vi "Replace Constant in VI (Scalar).vi"(8 "error in":errorcluster, 10 "Constant Replacement Params":T1, 11 "Original VI":path=path "C:/Users/OneEd/OneDrive/Desktop/MicroPort Job/CTDB/src/db_script/DB Select Template.vi") -> (0 "error out":errorcluster, 3 "Save as out":path=path "C:/Users/OneEd/OneDrive/Desktop/MicroPort Job/CTDB/src/db_script/DB Select Template.vi")   [LabVIEW 2021, in "EDT VI Script.lvlib"]
uses:
  EDT VI Script.lvlib
  Constant Replacement Param.ctl
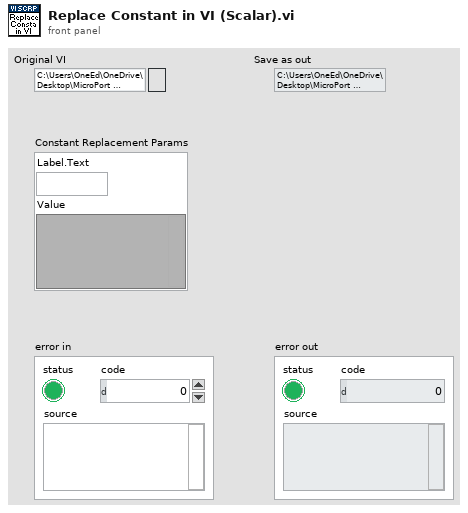
[diagram p1: front panel]
types:
  T1 = typedef "EDT VI Script.lvlib/Constant Replacement Param.ctl" = cluster{"Label.Text":string, "Value":variant}
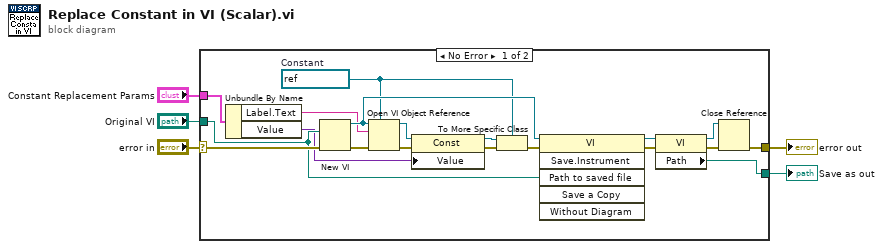
[diagram p0: block diagram]
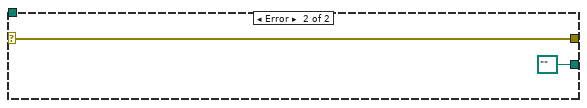
[diagram p2: hidden frame]
diagram:
  n1 = case shown="No Error" "error in" {
    selector: "error in" -> [w24 w26]
    tunnel: [w22 w26] -> w4
    tunnel: "Original VI" -> [w15 _]
    tunnel: [w18 path "" ("Path")] -> w2
    tunnel: "Constant Replacement Params" -> [w14 _]
    frame No Error {
      w6 = refnum<vi> refnum  # Constant
      n2 = Unbundle By Name(w14) -> ("Label.Text"=w8:string, "Value"=w7:variant)
      n3 = New VI(8:w24, 10:w15) -> (0:w23:errorcluster, 3:w21:refnum<vi>)  [unwired: 5 in]
      n4 = Open VI Object Reference(7:w6, 8:w23, 10:w8, 11:w21) -> (0:w11:errorcluster, 3:w12:refnum<vi>)
      n5 = property class="Const"(reference=w12, error in=w11, "Value"=w7) -> (reference out=w10:refnum<vi>, error out=w9:errorcluster)
      n6 = To More Specific Class(target class=w6, reference=w10, error in=w9) -> (error out=w13:errorcluster)  [unwired: 1 out]
      n7 = invoke class="VI" method="Save.Instrument"(reference=w21, error in=w13, "Path to saved file"=w15) -> (reference out=w17:refnum<vi>, error out=w16:errorcluster)  [unwired: 3 in, 4 out]
      n8 = property class="VI"(reference=w17, error in=w16) -> (reference out=w20:refnum<vi>, error out=w19:errorcluster, "Path"=w18:path)
      n9 = Close Reference(reference=w20, error in (no error)=w19) -> (error out=w22:errorcluster)
    }
    frame Error {
    }
  }
  "error out" <- w4
  "Save as out" <- w2
